vi "listen_port_10ms.vi"(8 "error in (no error)":errorcluster, 11 "canon_m3 in":refnum<class "protocol_canonM3.lvclass">) -> (0 "error out":errorcluster, 3 "canon_m3 out":refnum<class "protocol_canonM3.lvclass">)   [LabVIEW 2015, in "protocol_canonM3.lvclass"]
uses:
  protocol_canonM3.lvclass
  protocol_canonM3.lvclass/protocol_canonM3.ctl
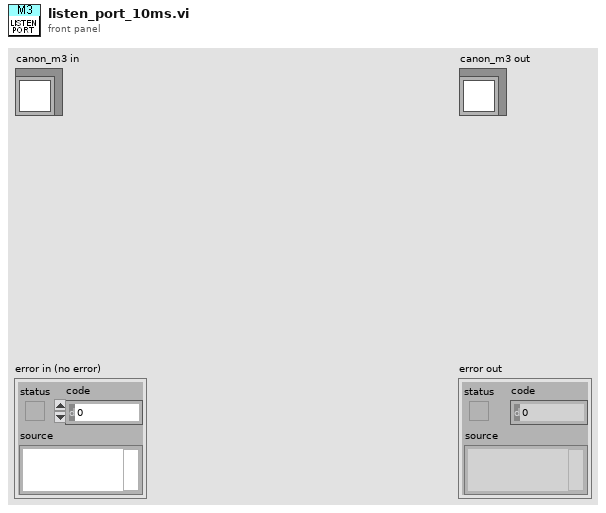
[diagram p1: front panel]
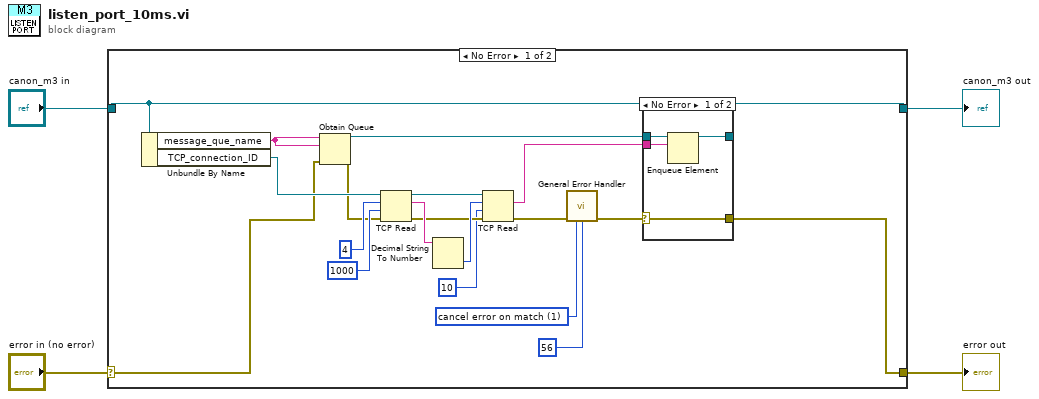
[diagram p0: block diagram]
diagram:
  n1 = case shown="No Error" "error in (no error)" {
    selector: "error in (no error)" -> [w11 w31]
    tunnel: [w5 w31] -> w3
    tunnel: [w23 w30] -> w1
    tunnel: "canon_m3 in" -> [w23 w30]
    frame No Error {
      w9 = 1 items=["no exception", "cancel error on match", "set error on match"] ("[exception action] (none:0)")
      n2 = Unbundle By Name(w23) -> ("message_que_name"=w14:string, "TCP_connection_ID"=w12:refnum<k5>)
      n3 = Obtain Queue(name (unnamed)=w14, element data type=w14, error in (no error)=w11) -> (queue out=w13:refnum<queue>, error out=w10:errorcluster)  [unwired: 2 in, 1 out]
      n4 = TCP Read(connection ID=w12, bytes to read=4, error in (no error)=w10, 9:1000 ("timeout ms (25000)")) -> (connection ID out=w17:refnum<k5>, data out=w20:string, error out=w18:errorcluster)  [unwired: 1 in]
      n5 = Decimal String To Number(string=w20) -> (number=w19:i32)  [unwired: 2 in, 1 out]
      n6 = TCP Read(connection ID=w17, bytes to read=w19, error in (no error)=w18, 9:10 ("timeout ms (25000)")) -> (data out=w15:string, error out=w7:errorcluster)  [unwired: 1 in, 1 out]
      n7 = call <vilib>:"General Error Handler.vi"("error in (no error)"=w7, "[exception action] (none:0)"=w9, "[exception code]"=56) -> ("error out"=w6:errorcluster)  [unwired: 8 in, 4 out]
      n8 = case shown="No Error" w6 {
        selector: w6 -> [w24 w28]
        tunnel: w13 -> [w27 w29]
        tunnel: w15 -> [w26 _]
        tunnel: [w25 w29] -> _
        tunnel: [w24 w28] -> w5
        frame No Error {
          n9 = Enqueue Element(queue=w27, element=w26) -> (queue out=w25:refnum<queue>)  [unwired: 2 in, 2 out]
        }
        frame Error {
        }
      }
    }
    frame Error {
    }
  }
  "error out" <- w3
  "canon_m3 out" <- w1
